vi "Get Next Event Log Entry.vi"(8 "error in (no error)":errorcluster {"code" format="%.0x"}, 9 "LogEntryBufferSize":i32=256 caption="LogEntryBufferSize (256)", 11 "instrument handle":refnum<k15>) -> (0 "error out":errorcluster {"code" format="%.0x"}, 2 "LogEntry":string, 3 "instrument handle out":refnum<k15>)   [LabVIEW 2009, in "Keysight XSAn.lvlib"]
doc: "This VI retrieves and clears the oldest event log entry for the IVI session.\n\nSupported Models: N9000A, N9000B, N9010A, N9010B, N9020A, N9020B, N9030A, N9030B, N9038A, SPN9003A, SPN9026A"
uses:
  <instrlib>/Keysight XSAn/Keysight XSAn.lvlib
  AgXSAn.dll
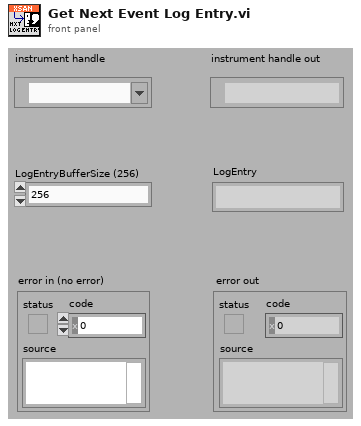
[diagram p1: front panel]
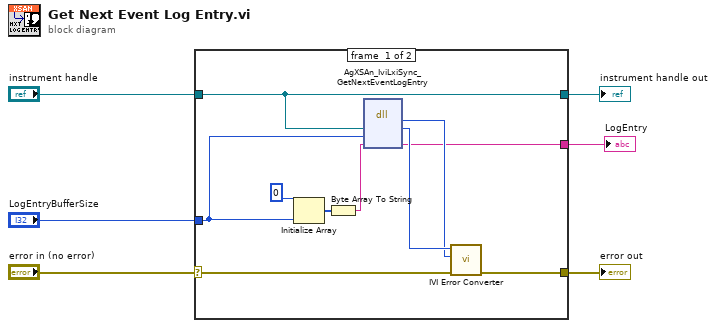
[diagram p0: block diagram]
diagram:
  n1 = case shown="No Error" "error in (no error)" {
    selector: "error in (no error)" -> [w14 w18]
    tunnel: [w13 w18] -> w6
    tunnel: "instrument handle" -> [w8 w17]
    tunnel: "LogEntryBufferSize" -> [w7 _]
    tunnel: [w9 _] -> w2
    tunnel: [w8 w17] -> w1
    frame #0 {
      n2 = Initialize Array(u8 0 ("element"), w7) -> (w11:u8[])
      n3 = Byte Array To String(unsigned byte array=w11) -> (string=w12:string)
      n4 = dll-call lib="AgXSAn**.dll" fn="AgXSAn_IviLxiSync_GetNextEventLogEntry"("Vi"=w8, "LogEntryBufferSize"=w7, "LogEntry"=w12) -> (w15:i32, "Vi"=w16:u32, "LogEntry"=w9:string)  [unwired: 4 in, 2 out]
      n5 = call <instrlib>:"IVI Error Converter.vi"("error in (no error)"=w14, "IVI error code (0)"=w15, "instrument handle"=w16) -> ("error out"=w13:errorcluster)  [unwired: 7 in, 1 out]
    }
    frame #1 {
    }
  }
  "error out" <- w6
  "instrument handle out" <- w1
  "LogEntry" <- w2
